vi "Handle Error.vi"(8 "error in (no error)":errorcluster, 11 "CS++GoBangClient in":refnum<class "CS++GoBangClient.lvclass">) -> (0 "error out":errorcluster, 2 "stop actor?":bool=TRUE, 3 "CS++GoBangClient out":refnum<class "CS++GoBangClient.lvclass">)   [LabVIEW 2014, in "GoBang.lvlib" / "CS++GoBangClient.lvclass"]
doc: "(<B>Filename</B>: Actor Framework.lvlib:Actor.lvclass:Handle Error.vi)\n\nDefines how the actor handles an error that occurred while processing a message. By default, this method does nothing except stop the actor."
uses:
  CS++GoBangClient.lvclass
  CS++GoBangClient.lvclass/CS++GoBangClient.ctl
  <vilib>/ActorFramework/Actor/Actor.lvclass
  <vilib>/NI/Actors/Linked Network Actor/Linked Network Actor Messages/Connect Msg/Connect Msg.lvclass
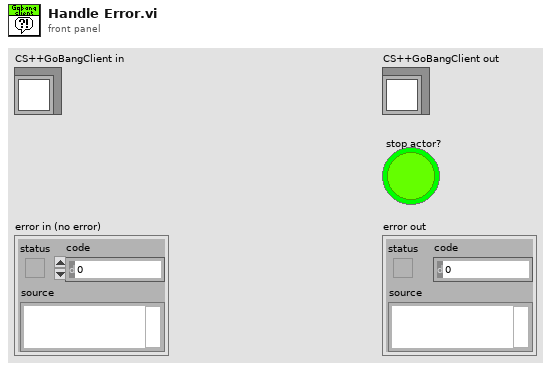
[diagram p1: front panel]
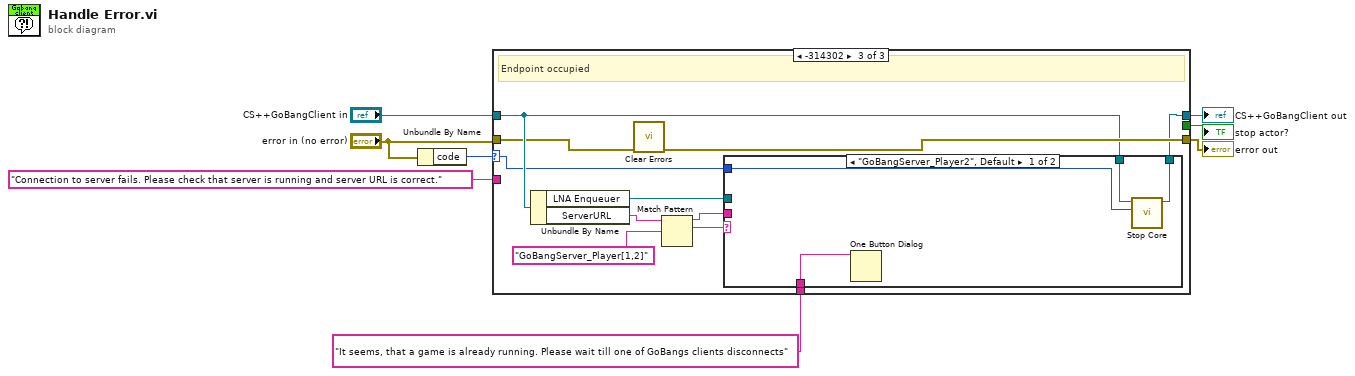
[diagram p0: block diagram]
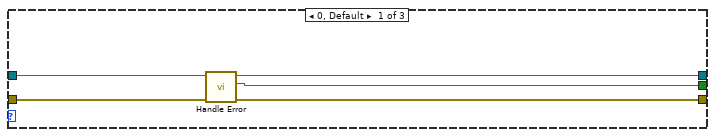
[diagram p2: hidden frame]
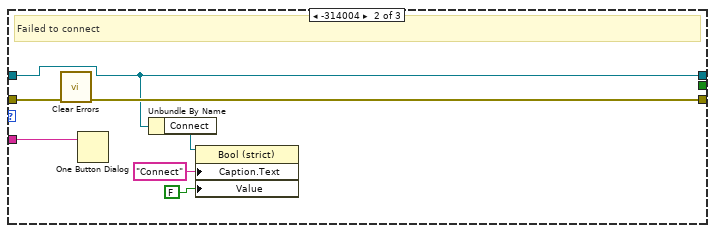
[diagram p3: hidden frame]
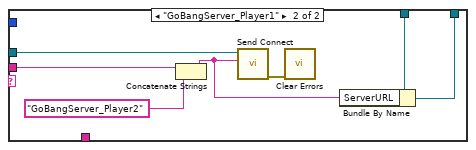
[diagram p4: hidden frame]
diagram:
  n1 = Unbundle By Name("error in (no error)") -> ("code"=w7:i32)
  n2 = case shown="-314302" w7 {
    selector: w7 -> [_ _ w21]
    tunnel: [w9 w19 w31] -> w3
    tunnel: "error in (no error)" -> [w10 w20 w22]
    tunnel: "Connection to server fails. Please check that server is running and server URL is correct." ("message") -> [_ w18 _]
    tunnel: "CS++GoBangClient in" -> [w13 w16 w24]
    tunnel: [w12 w16 w23] -> w4
    tunnel: [w11 _ _] -> w2
    tunnel: "It seems, that a game is already running. Please wait till one of GoBangs clients disconnects" ("message") -> [_ _ w30]
    frame 0, Default {
      n3 = call-parent "Handle Error.vi"("error in (no error)"=w10, "Actor in"=w13) -> ("error out"=w9:errorcluster, "stop actor?"=w11:bool, "Actor out"=w12:refnum<class "CS++GoBangClient.lvclass">)  [unwired: 7 in]
    }
    frame -314004 {
      # "Failed to connect"
      n4 = call <vilib>:"Clear Errors.vi"("error in (no error)"=w20) -> ("error out"=w19:errorcluster)  [unwired: 5 in, 1 out]
      n5 = One Button Dialog(message=w18) -> ()  [unwired: 1 in, 1 out]
      n6 = Unbundle By Name(w16) -> ("Connect"=w15:refnum<vi>)
      n7 = property class="Bool (strict)"(reference=w15, "Caption.Text"="Connect" ("Label.Text"), "Value"=FALSE) -> ()  [unwired: 1 in, 2 out]
    }
    frame -314302 {
      # "Endpoint occupied"
      n8 = Unbundle By Name(w24) -> ("LNA Enqueuer"=w29:refnum<class "Message Enqueuer.lvclass">, "ServerURL"=w27:string)
      n9 = call <vilib>:"Clear Errors.vi"("error in (no error)"=w22) -> ("error out"=w31:errorcluster)  [unwired: 5 in, 1 out]
      n10 = Match Pattern(string=w27, regular expression="GoBangServer_Player[1,2]") -> (before substring=w25:string, match substring=w28:string)  [unwired: 1 in, 2 out]
      n11 = case shown="\"GoBangServer_Player2\", Default" w28 {
        tunnel: w30 -> [w35 _]
        tunnel: w29 -> [_ w42]
        tunnel: w25 -> [_ w39]
        tunnel: w24 -> [w34 w38]
        tunnel: [w33 w37] -> w23
        tunnel: w21 -> [w32 _]
        frame "GoBangServer_Player2", Default {
          n12 = One Button Dialog(message=w35) -> ()  [unwired: 1 in, 1 out]
          n13 = call-dynamic "Stop Core.vi"("final error code"=w32, "CS++GoBangClient in"=w34) -> ("CS++GoBangClient out"=w33:refnum<class "CS++GoBangClient.lvclass">)  [unwired: 9 in]
        }
        frame "GoBangServer_Player1" {
          n14 = Concatenate Strings(w39, "GoBangServer_Player2" ("regular expression")) -> (w36:string)
          n15 = call <vilib>:"Send Connect.vi"("URL"=w36, "Message Enqueuer"=w42) -> ("error out"=w41:errorcluster)  [unwired: 8 in, 1 out]
          n16 = call <vilib>:"Clear Errors.vi"("error in (no error)"=w41) -> ()  [unwired: 5 in, 2 out]
          n17 = Bundle By Name(cluster=w38, "ServerURL"=w36) -> (w37:refnum<class "CS++GoBangClient.lvclass">)
        }
      }
    }
  }
  "CS++GoBangClient out" <- w4
  "error out" <- w3
  "stop actor?" <- w2
